vi "Create Server.vi"(8 "error in (no error)":errorcluster) -> (0 "error out":errorcluster, 3 "gRPCid":T1)   [LabVIEW 2019, in "ctet_dio.lvlib" / "gprc-lvsupport.lvlib"]
uses:
  gprc-lvsupport.lvlib
  typeDefs/grpcId.ctl
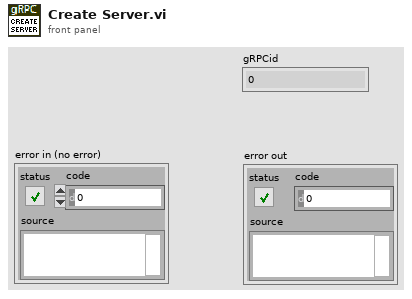
[diagram p1: front panel]
types:
  T1 = typedef "ctet_dio.lvlib/gprc-lvsupport.lvlib/grpcId.ctl" = u64
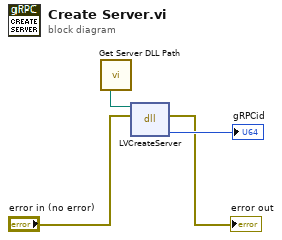
[diagram p0: block diagram]
diagram:
  n1 = call "Get Server DLL Path.vi"() -> ("Server dll path"=w1:path)
  n2 = dll-call lib="C:/Users/XEnderMD/Desktop/LV gRPC/labview source/gRPC interface/dlls/labview_grpc_server.dll" fn="LVCreateServer"(path in=w1, error in="error in (no error)") -> (error out=→"error out":errorcluster, "gRPCid"=→"gRPCid":T1)  [unwired: 3 in, 1 out]
